vi "倒计时.vi"() -> ()   [LabVIEW 2017]
panel:
  out "?":bool
  in  "开始倒计时":bool
  out "倒计时":timestamp format="%<%M:%S>T"
  in  "停止":bool
  in  "定时时间选择":enum16{"20秒", "10秒", "6秒"}(ring)
  # "倒计时器"
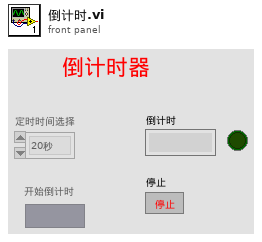
[diagram p1: front panel]
types:
  T1 = enum8{"Enabled", "Disabled", "Disabled and Grayed Out"}
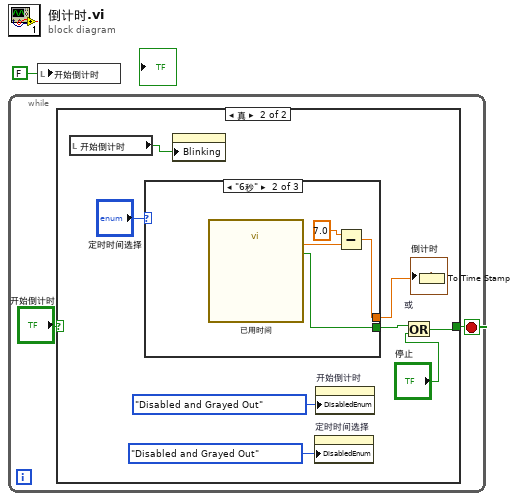
[diagram p0: block diagram]
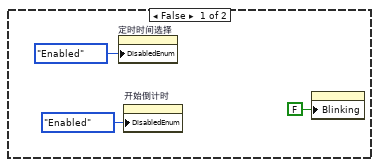
[diagram p2: hidden frame]
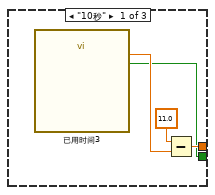
[diagram p3: hidden frame]
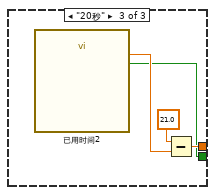
[diagram p4: hidden frame]
diagram:
  n1 = while {
    stop <- w3 stop-if-true
    n2 = case shown="真" "开始倒计时" {
      tunnel: [_ w12] -> w3
      frame False {
        n3 = property on="定时时间选择" class="Enum (严格)"("DisabledEnum"=T1."Enabled" ("禁用")) -> ()  [unwired: 2 in, 2 out]
        n4 = property on="开始倒计时" class="Bool (严格)"("DisabledEnum"=T1."Enabled" ("禁用")) -> ()  [unwired: 2 in, 2 out]
        n5 = property class="Bool (严格)"("Blinking"=FALSE ("闪烁")) -> ()  [unwired: 2 in, 2 out]
      }
      frame True {
        n6 = local read "开始倒计时"() -> (w10:bool)
        n7 = case shown="\"6秒\"" "定时时间选择" {
          tunnel: [w17 w21 w25] -> w8
          tunnel: [w16 w20 w24] -> w7
          frame "10秒" {
            n8 = call "已用时间3"() -> ("Elapsed Time (s)"=w19:dbl, "Time has Elapsed"=w16:bool)  [unwired: 12 in, 6 out]
            n9 = Subtract(x=11.0, y=w19) -> (x-y=w17:dbl)
          }
          frame "6秒" {
            n10 = call "已用时间"() -> ("Elapsed Time (s)"=w22:dbl, "Time has Elapsed"=w20:bool)  [unwired: 12 in, 6 out]
            n11 = Subtract(x=7.0, y=w22) -> (x-y=w21:dbl)
          }
          frame "20秒" {
            n12 = call "已用时间2"() -> ("Elapsed Time (s)"=w26:dbl, "Time has Elapsed"=w24:bool)  [unwired: 12 in, 6 out]
            n13 = Subtract(x=21.0, y=w26) -> (x-y=w25:dbl)
          }
        }
        n14 = property class="Bool (严格)"("Blinking"=w10) -> ()  [unwired: 2 in, 2 out]
        n15 = property on="定时时间选择" class="Enum (严格)"("DisabledEnum"=T1."Disabled and Grayed Out" ("禁用")) -> ()  [unwired: 2 in, 2 out]
        n16 = property on="开始倒计时" class="Bool (严格)"("DisabledEnum"=T1."Disabled and Grayed Out" ("禁用")) -> ()  [unwired: 2 in, 2 out]
        n17 = Or "或"(x=w7, y="停止") -> (x .or. y?=w12:bool)
        n18 = To Time Stamp(1:w8) -> (0:→"倒计时":timestamp)
      }
    }
  }
  n19 = local write "开始倒计时"(FALSE) -> ()
